vi "Main1.vi"() -> ()   [LabVIEW 2014]
uses:
  Control/Control_process.ctl
  Program Files (x86)/National Instruments/LabVIEW 2018/instr.lib/OSICS 1.1.0/OSICS_LIB.lvlib
  <vilib>/Utility/file.llb/Write Delimited Spreadsheet (string).vi
panel:
  in  "Ref_spec Button":bool
  in  "WL_delay(ms)":u32=800
  in  "Read Button":bool
  in  "VISA_PWM":refnum<visa-resource-name> caption="Power Meter"
  in  "VISA_TLS":refnum<visa-resource-name> caption="Light Source"
  in  "WL_Set":dbl=1310.0 caption="Wavelength"
  in  "PM_delay(ms)":i32=200
  in  "Link Button":bool
  in  "WL_step":dbl=1.0 caption="Step(nm)"
  out "pow_read":dbl caption="Pow"
  in  "Unit(dB:T)":bool
  out "REF?":bool caption="Single Ref."
  out "testing?":bool caption="Bussy"
  out "link?":bool caption="Eq. Online"
  out "Msg":string
  in  "Stop Button":bool
  in  "Sweep Button":bool
  in  "Ref Button":bool
  out "pow_chart":dbl(graph)
  out "WL_Peak":dbl caption="Peak"
  in  "WL_End":dbl=1350.0 caption="End(nm)"
  in  "WL_Start":dbl=1260.0 caption="Start(nm)"
  # "ADDR."
  # "READ"
  # "SWEEP"
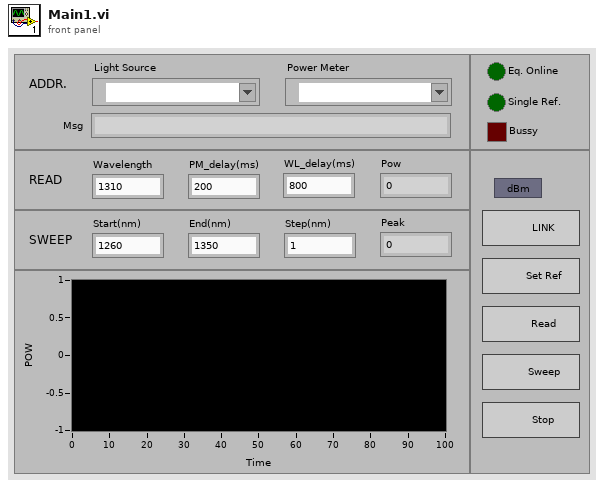
[diagram p1: front panel]
types:
  T1 = typedef "Control_process.ctl" = enum16{"init", "link", "reference", "reference2", "wave_chng", "lockpanel", "single", "sweep", "log_res", "quit"}
  T2 = cluster{"Laser State":bool, "WL/F Value":dbl, "Power (dBm/mW)":dbl, "Power Limit":bool}
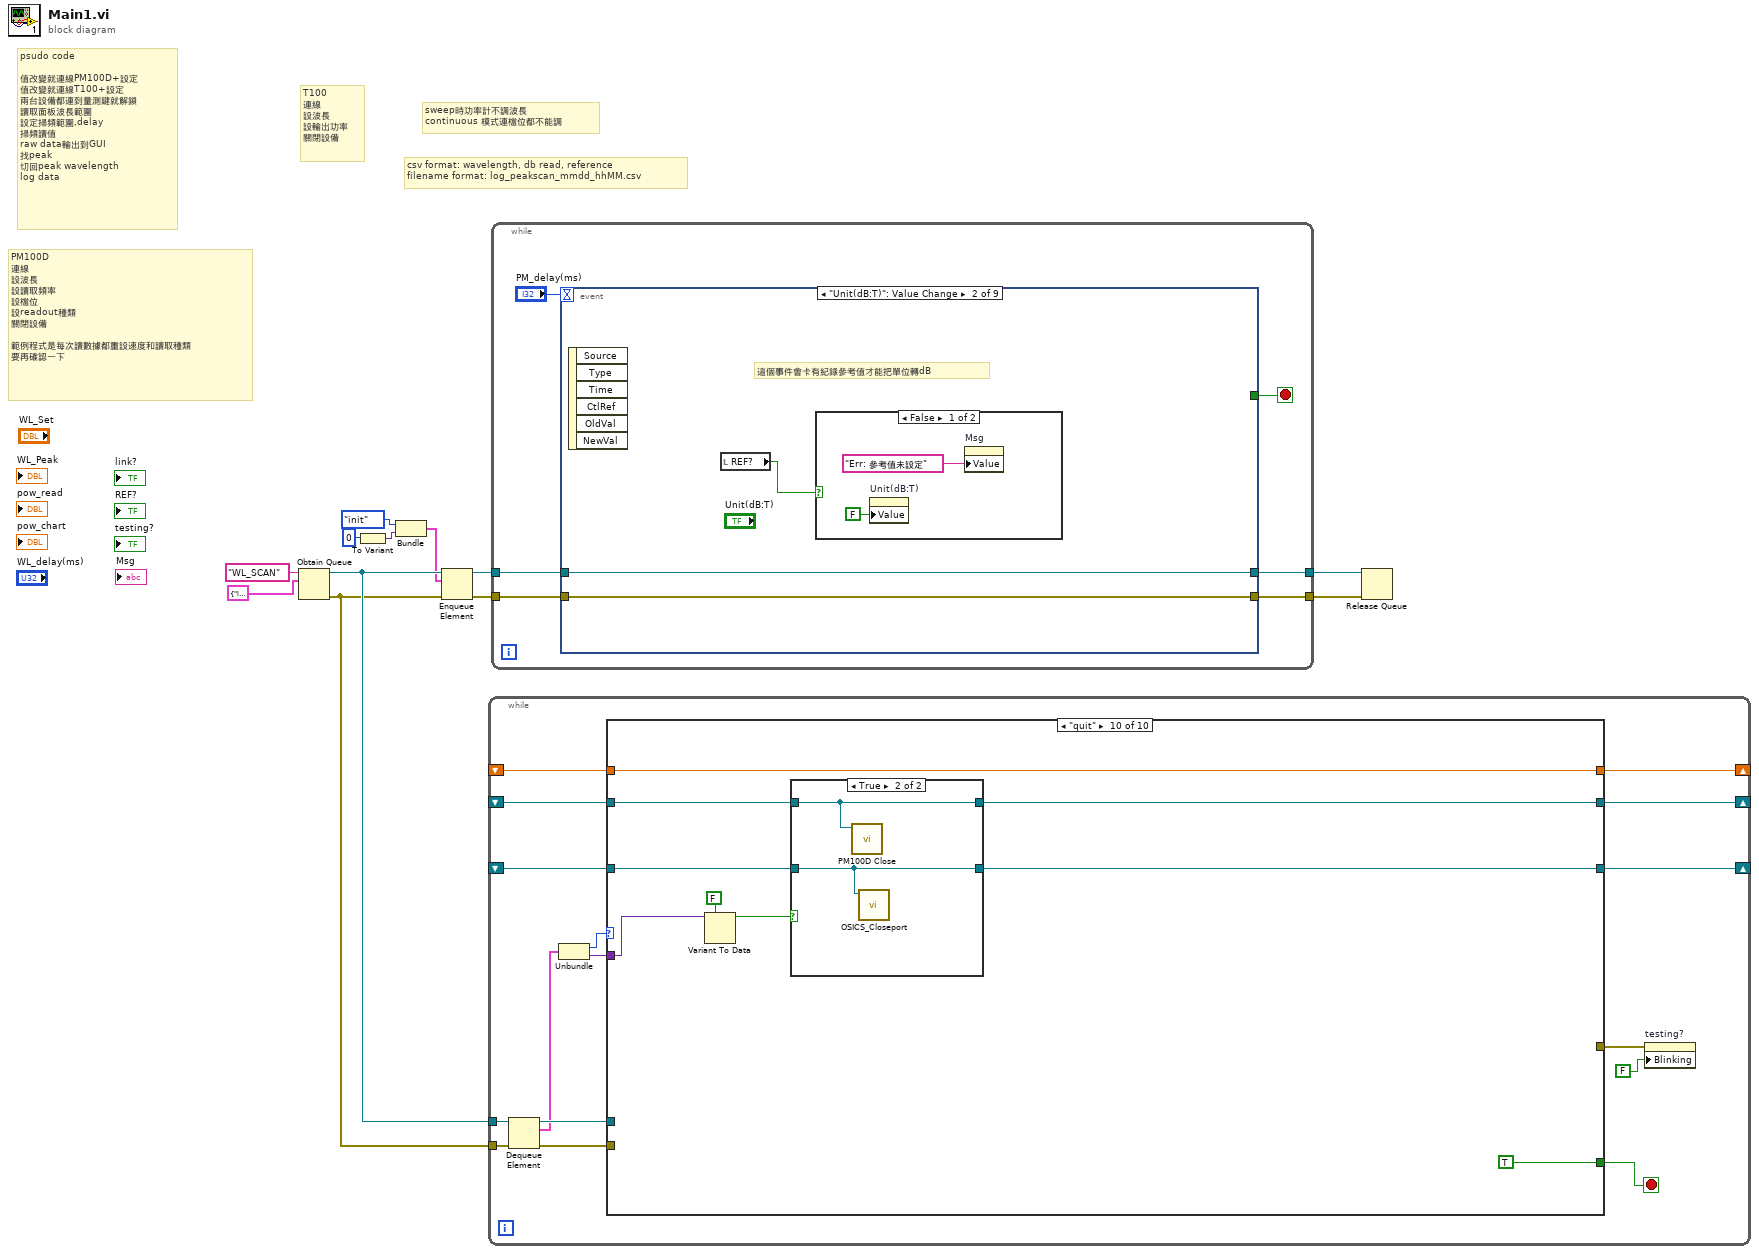
[diagram p0: block diagram]
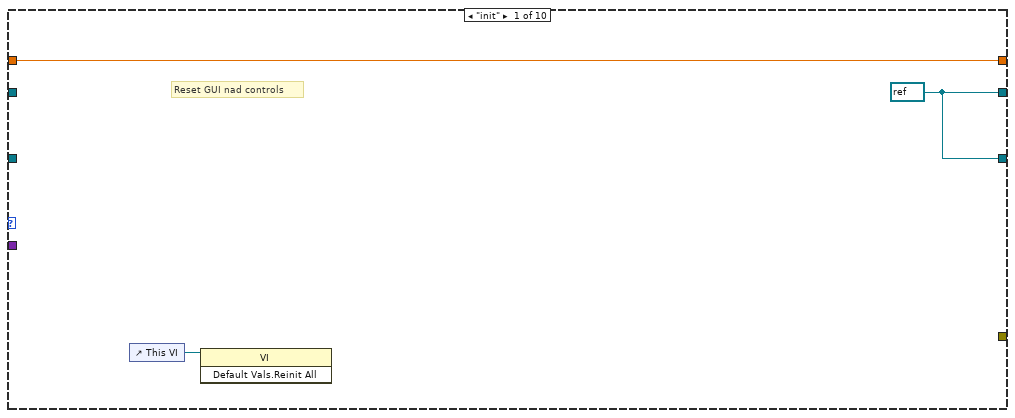
[diagram p2: hidden frame]
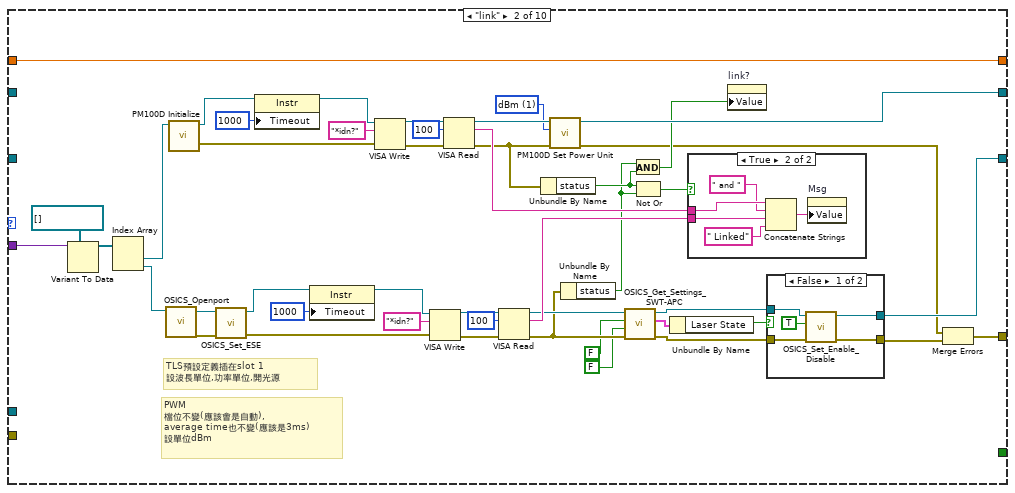
[diagram p3: hidden frame]
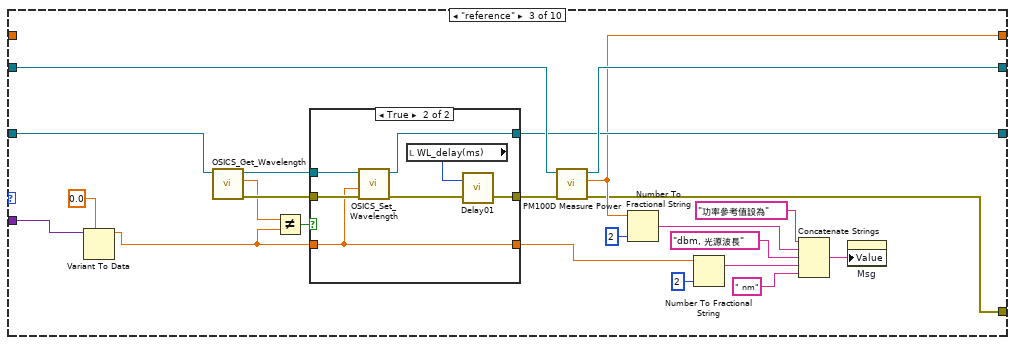
[diagram p6: hidden frame]
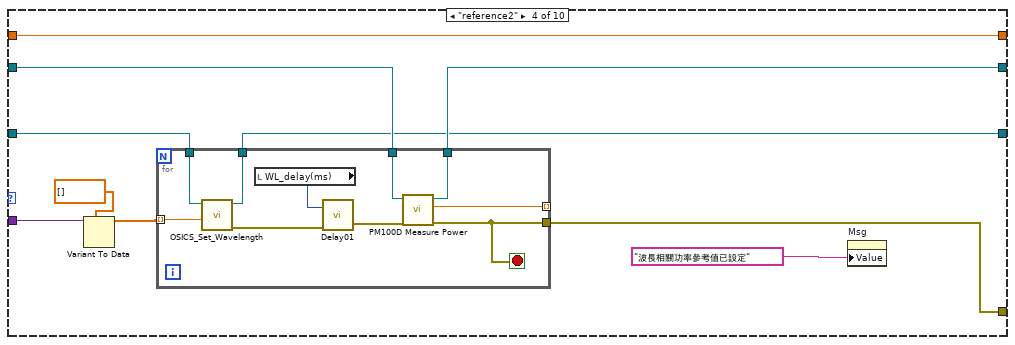
[diagram p8: hidden frame]
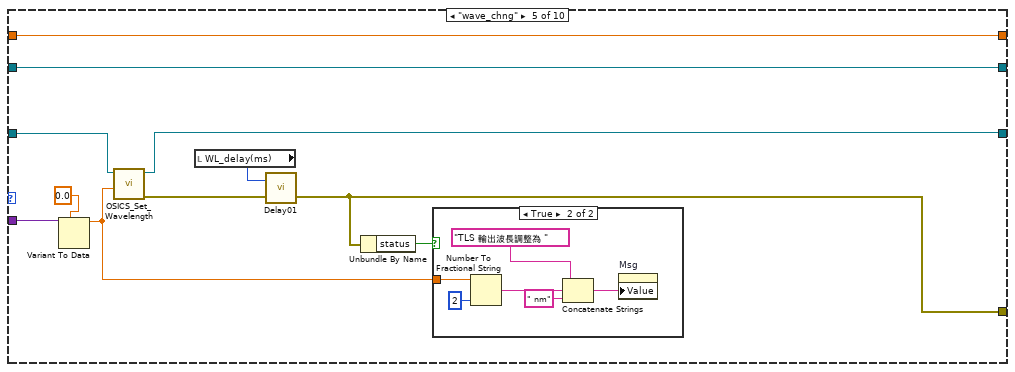
[diagram p9: hidden frame]
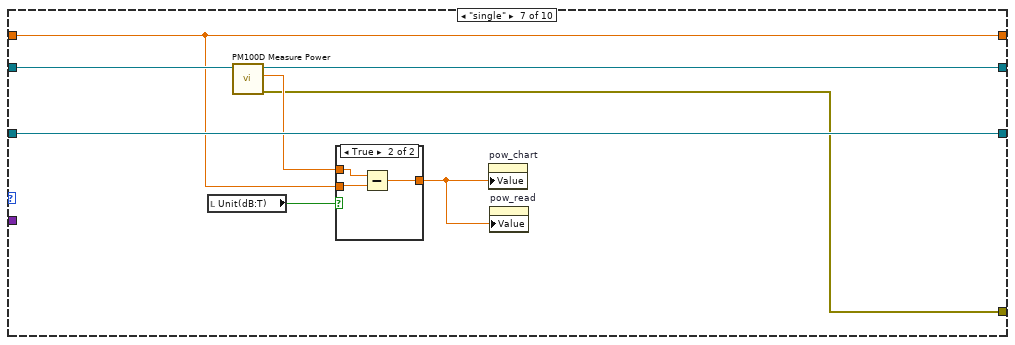
[diagram p12: hidden frame]
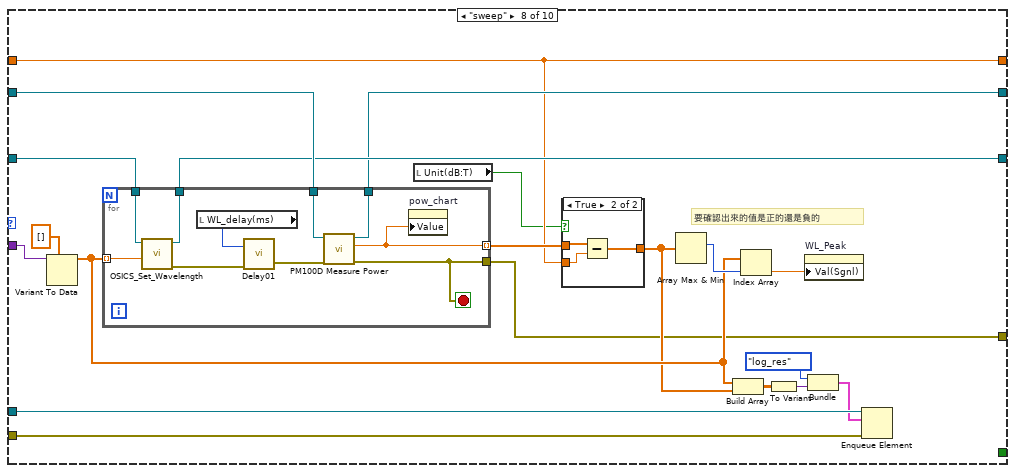
[diagram p14: hidden frame]
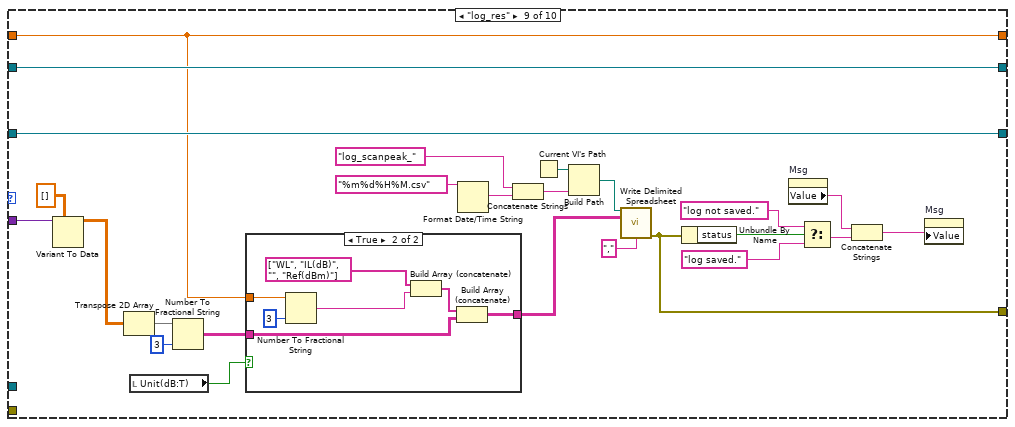
[diagram p16: hidden frame]
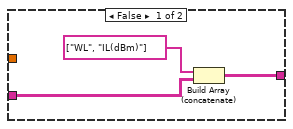
[diagram p17: hidden frame]
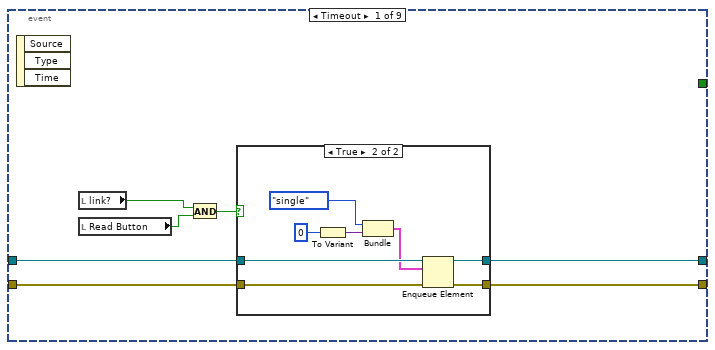
[diagram p19: hidden frame]
diagram:
  # "csv format: wavelength, db read, reference\nfilename format: log_peakscan_mmdd_hhMM.csv"
  # "sweep時功率計不調波長\ncontinuous 模式連檔位都不能調"
  # "T100\n連線\n設波長\n設輸出功率\n關閉設備"
  # "PM100D\n連線\n設波長\n設讀取頻率\n設檔位\n設readout種類\n關閉設備\n\n範例程式是每次讀數據都重設速度和讀取種類\n要再確認一下"
  # "psudo code\n\n值改變就連線PM100D+設定\n值改變就連線T100+設定\n兩台設備都連到量測鍵就解鎖\n讀取面板波長範圍\n設定掃頻範圍,delay\n掃頻讀值\nraw data輸出到GUI\n找peak\n切回peak wavelength\nlog data"
  n1 = Obtain Queue(name (unnamed)="WL_SCAN", element data type=cluster{"Proc":T1, variant} {"Proc"=enum."init", variant}) -> (queue out=w11:refnum<queue>, error out=w6:errorcluster)  [unwired: 3 in, 1 out]
  n2 = To Variant(anything=0) -> (Variant=w3:variant)
  n3 = Bundle("Proc"=Control_process."init", "Variant"=w3) -> (w1:cluster{"Proc":T1, "Variant":variant})  [unwired: 1 in]
  n4 = Enqueue Element(queue=w11, element=w1, error in (no error)=w6) -> (queue out=w7:refnum<queue>, error out=w5:errorcluster)  [unwired: 1 in, 1 out]
  n5 = while {
    tunnel: w6 -> [w26]
    tunnel: w11 -> [w28]
    shift-right: [w17] -> _
    shift-left: _ -> [w21]
    shift-right: [w20] -> _
    shift-left: _ -> [w19]
    shift-right: [w14] -> _
    shift-left: _ -> [w13]
    stop <- w18 stop-if-true
    n6 = Dequeue Element(queue=w28, error in (no error)=w26) -> (queue out=w27:refnum<queue>, element=w24:cluster{"Proc":T1, variant}, error out=w25:errorcluster)  [unwired: 1 in, 1 out]
    n7 = Unbundle(w24) -> ("Proc"=w23:T1, w22:variant)
    n8 = case shown="\"quit\"" w23 {
      tunnel: w27 -> [_ _ _ _ _ _ _ w186 _ _]
      tunnel: w25 -> [_ _ _ _ _ _ _ w185 _ _]
      tunnel: w22 -> [_ w77 w110 w132 w151 _ _ w193 w232 w247]
      tunnel: w21 -> [_ _ w112 w127 w146 w161 w170 w194 w217 w250]
      tunnel: [w31 w43 w108 w125 w152 w160 w169 w192 w228 w248] -> w20
      tunnel: w19 -> [_ _ w106 w128 w153 w160 w169 w191 w228 w252]
      tunnel: [_ _ _ _ _ _ _ _ _ TRUE] -> w18
      tunnel: [w31 w39 w111 w126 w146 w161 w168 w180 w217 w249] -> w17
      tunnel: [_ w33 w92 w124 w143 _ w163 w175 w211 _] -> w15
      tunnel: [w29 w35 w96 w129 w144 w162 w166 w178 w210 w244] -> w14
      tunnel: w13 -> [w29 w35 _ w129 w144 w162 w166 w178 w210 w244]
      frame "init" {
        w31 = refnum<visa-resource-name> refnum ("instrument handle out")
        # "Reset GUI nad controls"
        n9 = control-ref of="This VI"() -> (w30:refnum<vi>)
        n10 = invoke class="VI" method="Default Vals.Reinit All"(reference=w30) -> ()  [unwired: 2 in, 3 out]
      }
      frame "link" {
        w41 = i16 1 items=["Watt", "dBm"] ("Power Unit (Watt)")
        # "TLS預設定義插在slot 1\n設波長單位,功率單位,開光源"
        # "PWM\n檔位不變(應該會是自動), \naverage time也不變(應該是3ms)\n設單位dBm"
        n11 = Variant To Data(type=refnum<visa-resource-name>[] [] ("appended array"), Variant=w77) -> (data=w75:refnum<visa-resource-name>[])  [unwired: 1 in, 1 out]
        n12 = Index Array(array=w75) -> (element #1=w74:refnum<visa-resource-name>, element #2=w64:refnum<visa-resource-name>)  [unwired: 2 in]
        n13 = call "OSICS_Openport.vi"("VISA IN"=w64) -> ("error out"=w65:errorcluster, "VISA OUT"=w63:refnum<visa-resource-name>)  [unwired: 9 in]
        n14 = call "PM100D Initialize.vi"("resource name"=w74) -> ("error out"=w69:errorcluster, "instrument handle out"=w68:refnum<visa-resource-name>)  [unwired: 9 in]
        n15 = call "OSICS_Set_ESE.vi"("error in (no error)"=w65, "VISA resource name"=w63) -> ("error out"=w56:errorcluster, "VISA resource name out"=w55:refnum<visa-resource-name>)  [unwired: 8 in]
        n16 = property class="Instr"(reference=w68, "Timeout"=u32 1000 ("General Settings:Timeout Value")) -> (reference out=w67:refnum<visa-resource-name>)  [unwired: 1 in, 1 out]
        n17 = property class="Instr"(reference=w55, "Timeout"=u32 1000 ("General Settings:Timeout Value")) -> (reference out=w61:refnum<visa-resource-name>)  [unwired: 1 in, 1 out]
        n18 = VISA Write(VISA resource name=w67, write buffer="*idn?", error in (no error)=w69) -> (VISA resource name out=w71:refnum<visa-resource-name>, error out=w73:errorcluster)  [unwired: 1 out]
        n19 = VISA Write(VISA resource name=w61, write buffer="*idn?", error in (no error)=w56) -> (VISA resource name out=w59:refnum<visa-resource-name>, error out=w57:errorcluster)  [unwired: 1 out]
        n20 = VISA Read(VISA resource name=w71, byte count=u32 100, error in (no error)=w73) -> (VISA resource name out=w42:refnum<visa-resource-name>, read buffer=w53:string, error out=w40:errorcluster)  [unwired: 1 out]
        n21 = VISA Read(VISA resource name=w59, byte count=u32 100, error in (no error)=w57) -> (VISA resource name out=w51:refnum<visa-resource-name>, read buffer=w54:string, error out=w48:errorcluster)  [unwired: 1 out]
        n22 = Unbundle By Name(w40) -> ("status"=w37:bool)
        n23 = call "PM100D Set Power Unit.vi"("error in (no error)"=w40, "Power Unit (Watt)"=w41, "instrument handle"=w42) -> ("error out"=w32:errorcluster, "instrument handle out"=w39:refnum<visa-resource-name>)  [unwired: 7 in]
        n24 = Unbundle By Name(w48) -> ("status"=w36:bool)
        n25 = call "OSICS_Get_Settings_SWT-APC.vi"("error in"=w48, "Power Unit(dBm/mW)"=FALSE, "WL/F unit (nm/GHz)"=FALSE, "VISA IN"=w51) -> ("error out"=w44:errorcluster, "Laser Settings (Cluster)"=w50:T2, "VISA OUT"=w45:refnum<visa-resource-name>)  [unwired: 5 in]
        n26 = And(x=w36, y=w37) -> (x .and. y?=w38:bool)
        n27 = Not Or(1:w36, 2:w37) -> (0:w52:bool)
        n28 = Unbundle By Name(w50) -> ("Laser State"=w49:bool)
        n29 = case shown="True" w52 {
          tunnel: w54 -> [_ w89]
          tunnel: w53 -> [_ w88]
          frame False {
          }
          frame True {
            n30 = Concatenate Strings(w88, " and " ("string"), w89, " Linked" ("string")) -> (w86:string)
            n31 = property on="Msg" class="Str"("Value"=w86) -> ()  [unwired: 2 in, 2 out]
          }
        }
        n32 = property on="link?" class="Bool (strict)"("Value"=w38) -> ()  [unwired: 2 in, 2 out]
        n33 = case shown="False" w49 {
          tunnel: w45 -> [w81 w84]
          tunnel: w44 -> [w80 w83]
          tunnel: [w79 w84] -> w43
          tunnel: [w78 w83] -> w34
          frame False {
            n34 = call "OSICS_Set_Enable_Disable.vi"("error in"=w80, "Laser State (False:DISABLED)"=TRUE, "VISA IN"=w81) -> ("error out"=w78:errorcluster, "VISA OUT"=w79:refnum<visa-resource-name>)  [unwired: 6 in, 1 out]
          }
          frame True {
          }
        }
        n35 = Merge Errors(w32, w34) -> (w33:errorcluster)
      }
      frame "reference" {
        n36 = Variant To Data(type=0.0, Variant=w110) -> (data=w90:dbl)  [unwired: 1 in, 1 out]
        n37 = call "OSICS_Get_Wavelength.vi"("VISA IN"=w106) -> ("error out"=w105:errorcluster, "WL/Frequency Value"=w103:dbl, "VISA OUT"=w107:refnum<visa-resource-name>)  [unwired: 7 in, 1 out]
        n38 = Not Equal?(x=w103, y=w90) -> (x != y?=w104:bool)
        n39 = case shown="True" w104 {
          tunnel: [w114 w120] -> w109
          tunnel: [w115 w119] -> w108
          tunnel: w107 -> [w115 w118]
          tunnel: w105 -> [w114 w117]
          tunnel: w90 -> [w113 w116]
          tunnel: [w113 w116] -> w93
          frame False {
          }
          frame True {
            n40 = call "OSICS_Set_Wavelength.vi"("error in"=w117, "WL/Frequency Value"=w116, "VISA IN"=w118) -> ("error out"=w122:errorcluster, "VISA OUT"=w119:refnum<visa-resource-name>)  [unwired: 6 in, 1 out]
            n41 = local read "WL_delay(ms)"() -> (w121:u32)
            n42 = call "Delay01.vi"("error in"=w122, "ms delay"=w121) -> ("error out"=w120:errorcluster)  [unwired: 1 in]
          }
        }
        n43 = call "PM100D Measure Power.vi"("error in (no error)"=w109, "instrument handle"=w112) -> ("error out"=w92:errorcluster, "Power"=w96:dbl, "instrument handle out"=w111:refnum<visa-resource-name>)  [unwired: 7 in]
        n44 = Number To Fractional String(number=w96, precision (6)=i16 2) -> (F-format string=w95:string)  [unwired: 2 in]
        n45 = Number To Fractional String(number=w93, precision (6)=i16 2) -> (F-format string=w100:string)  [unwired: 2 in]
        n46 = Concatenate Strings("功率參考值設為" ("string"), w95, "dbm, 光源波長" ("string"), w100, " nm" ("string")) -> (w99:string)
        n47 = property on="Msg" class="Str"("Value"=w99) -> ()  [unwired: 2 in, 2 out]
      }
      frame "reference2" {
        n48 = Variant To Data(type=dbl[] [], Variant=w132) -> (data=w130:dbl[])  [unwired: 1 in, 1 out]
        n49 = for {
          tunnel: w127 -> [w142]
          tunnel: [w141] -> w126
          tunnel: [w138] -> w125
          tunnel: w128 -> [w137]
          tunnel: [w134] -> w124
          tunnel: [w136] -> _ mode=indexing
          tunnel: w130 -> [w135] mode=indexing
          stop <- w134 stop-if-true
          n50 = call "OSICS_Set_Wavelength.vi"("WL/Frequency Value"=w135, "VISA IN"=w137) -> ("error out"=w140:errorcluster, "VISA OUT"=w138:refnum<visa-resource-name>)  [unwired: 7 in, 1 out]
          n51 = local read "WL_delay(ms)"() -> (w133:u32)
          n52 = call "Delay01.vi"("error in"=w140, "ms delay"=w133) -> ("error out"=w139:errorcluster)  [unwired: 1 in]
          n53 = call "PM100D Measure Power.vi"("error in (no error)"=w139, "instrument handle"=w142) -> ("error out"=w134:errorcluster, "Power"=w136:dbl, "instrument handle out"=w141:refnum<visa-resource-name>)  [unwired: 7 in]
        }
        n54 = property on="Msg" class="Str"("Value"="波長相關功率參考值已設定" ("string")) -> ()  [unwired: 2 in, 2 out]
      }
      frame "wave_chng" {
        n55 = Variant To Data(type=0.0, Variant=w151) -> (data=w145:dbl)  [unwired: 1 in, 1 out]
        n56 = call "OSICS_Set_Wavelength.vi"("WL/Frequency Value"=w145, "VISA IN"=w153) -> ("error out"=w149:errorcluster, "VISA OUT"=w152:refnum<visa-resource-name>)  [unwired: 7 in, 1 out]
        n57 = local read "WL_delay(ms)"() -> (w147:u32)
        n58 = call "Delay01.vi"("error in"=w149, "ms delay"=w147) -> ("error out"=w143:errorcluster)  [unwired: 1 in]
        n59 = Unbundle By Name(w143) -> ("status"=w148:bool)
        n60 = case shown="True" w148 {
          tunnel: w145 -> [_ w156]
          frame False {
          }
          frame True {
            n61 = Number To Fractional String(number=w156, precision (6)=i16 2) -> (F-format string=w155:string)  [unwired: 2 in]
            n62 = Concatenate Strings("TLS 輸出波長調整為 " ("Msg"), w155, " nm" ("string")) -> (w159:string)
            n63 = property on="Msg" class="Str"("Value"=w159) -> ()  [unwired: 2 in, 2 out]
          }
        }
      }
      frame "lockpanel" {
      }
      frame "single" {
        n64 = local read "Unit(dB:T)"() -> (w164:bool)
        n65 = call "PM100D Measure Power.vi"("instrument handle"=w170) -> ("error out"=w163:errorcluster, "Power"=w167:dbl, "instrument handle out"=w168:refnum<visa-resource-name>)  [unwired: 8 in]
        n66 = case shown="True" w164 {
          tunnel: w167 -> [w171 w174]
          tunnel: w166 -> [_ w173]
          tunnel: [w171 w172] -> w165
          frame False {
          }
          frame True {
            n67 = Subtract(x=w174, y=w173) -> (x-y=w172:dbl)
          }
        }
        n68 = property on="pow_chart" class="WFChart (strict)"("Value"=w165) -> ()  [unwired: 2 in, 2 out]
        n69 = property on="pow_read" class="DigNum (strict)"("Value"=w165) -> ()  [unwired: 2 in, 2 out]
      }
      frame "sweep" {
        # "要確認出來的值是正的還是負的"
        n70 = Variant To Data(type=dbl[] [], Variant=w193) -> (data=w187:dbl[])  [unwired: 1 in, 1 out]
        n71 = for {
          tunnel: w194 -> [w208]
          tunnel: [w207] -> w180
          tunnel: [w203] -> w192
          tunnel: w191 -> [w202]
          tunnel: [w199] -> w175
          tunnel: [w201] -> w179 mode=indexing
          tunnel: w187 -> [w200] mode=indexing
          stop <- w199 stop-if-true
          n72 = call "OSICS_Set_Wavelength.vi"("WL/Frequency Value"=w200, "VISA IN"=w202) -> ("error out"=w206:errorcluster, "VISA OUT"=w203:refnum<visa-resource-name>)  [unwired: 7 in, 1 out]
          n73 = local read "WL_delay(ms)"() -> (w205:u32)
          n74 = call "Delay01.vi"("error in"=w206, "ms delay"=w205) -> ("error out"=w204:errorcluster)  [unwired: 1 in]
          n75 = call "PM100D Measure Power.vi"("error in (no error)"=w204, "instrument handle"=w208) -> ("error out"=w199:errorcluster, "Power"=w201:dbl, "instrument handle out"=w207:refnum<visa-resource-name>)  [unwired: 7 in]
          n76 = property on="pow_chart" class="WFChart (strict)"("Value"=w201) -> ()  [unwired: 2 in, 2 out]
        }
        n77 = local read "Unit(dB:T)"() -> (w176:bool)
        n78 = case shown="True" w176 {
          tunnel: w179 -> [w195 w198]
          tunnel: w178 -> [_ w197]
          tunnel: [w195 w196] -> w177
          frame False {
          }
          frame True {
            n79 = Subtract(x=w198, y=w197) -> (x-y=w196:dbl[])
          }
        }
        n80 = Array Max & Min(array=w177) -> (max index (indices)=w189:i32)  [unwired: 3 out]
        n81 = Build Array(w187, w177) -> (w182:dbl[][])
        n82 = Index Array(array=w187, index=w189) -> (element=w188:dbl)
        n83 = To Variant(anything=w182) -> (Variant=w183:variant)
        n84 = property on="WL_Peak" class="DigNum (strict)"("Val(Sgnl)"=w188) -> ()  [unwired: 2 in, 2 out]
        n85 = Bundle("Proc"=Control_process."log_res", "Variant"=w183) -> (w181:cluster{"Proc":T1, "Variant":variant})  [unwired: 1 in]
        n86 = Enqueue Element(queue=w186, element=w181, error in (no error)=w185) -> ()  [unwired: 1 in, 3 out]
      }
      frame "log_res" {
        n87 = Variant To Data(type=dbl[][] [] ("appended array"), Variant=w232) -> (data=w214:dbl[][])  [unwired: 1 in, 1 out]
        n88 = Transpose 2D Array(2D array=w214) -> (transposed array=w215:dbl[][])
        n89 = local read "Unit(dB:T)"() -> (w209:bool)
        n90 = Number To Fractional String(number=w215, precision (6)=i16 3) -> (F-format string=w213:string[][])  [unwired: 2 in]
        n91 = case shown="True" w209 {
          tunnel: w213 -> [w236 w243]
          tunnel: [w234 w242] -> w212
          tunnel: w210 -> [_ w239]
          frame False {
            n92 = Build Array (concatenate)(string[] ["WL", "IL(dBm)"], w236) -> (w234:string[][])
          }
          frame True {
            n93 = Number To Fractional String(number=w239, precision (6)=i16 3) -> (F-format string=w238:string)  [unwired: 2 in]
            n94 = Build Array (concatenate)(string[] ["WL", "IL(dB)", "", "Ref(dBm)"], w238) -> (w241:string[])
            n95 = Build Array (concatenate)(w241, w243) -> (w242:string[][])
          }
        }
        n96 = Format Date/Time String(time format string (%c)="%m%d%H%M.csv") -> (date/time string=w225:string)  [unwired: 2 in]
        n97 = Concatenate Strings("log_scanpeak_" ("string"), w225) -> (w224:string)
        n98 = Current VI's Path() -> (path=w230:path)
        n99 = Build Path(base path=w230, name or relative path=w224) -> (appended path=w229:path)
        n100 = call-poly <vilib>:"Write Delimited Spreadsheet.vi"("file path (dialog if empty)"=w229, "2D data"=w212, "delimiter (\\t)"="," ("delimiter (\\t)")) -> ("error out"=w211:errorcluster)  [unwired: 11 in, 1 out]
        n101 = Unbundle By Name(w211) -> ("status"=w223:bool)
        n102 = property on="Msg" class="Str"() -> ("Value"=w220:string)  [unwired: 2 in, 2 out]
        n103 = Select(t="log not saved.", s=w223, f="log saved.") -> (s? t:f=w221:string)
        n104 = Concatenate Strings(w220, w221) -> (w222:string)
        n105 = property on="Msg" class="Str"("Value"=w222) -> ()  [unwired: 2 in, 2 out]
      }
      frame "quit" {
        n106 = Variant To Data(type=FALSE, Variant=w247) -> (data=w245:bool)  [unwired: 1 in, 1 out]
        n107 = case shown="True" w245 {
          tunnel: w252 -> [w253 w255]
          tunnel: w250 -> [w254 w256]
          tunnel: [w254 w256] -> w249
          tunnel: [w253 w255] -> w248
          frame False {
          }
          frame True {
            n108 = call "PM100D Close.vi"("instrument handle"=w256) -> ()  [unwired: 10 in, 1 out]
            n109 = call "OSICS_Closeport.vi"("VISA IN"=w255) -> ()  [unwired: 10 in, 1 out]
          }
        }
      }
    }
    n110 = property on="testing?" class="Bool (strict)"(error in=w15, "Blinking"=FALSE) -> ()  [unwired: 1 in, 2 out]
  }
  n111 = while {
    tunnel: w7 -> [w260]
    tunnel: w5 -> [w261]
    tunnel: [w259] -> w10
    tunnel: [w258] -> w9
    stop <- w262 stop-if-true
    n112 = event shown="[1] \"Unit(dB:T)\": Value Change" {
      selector: _ -> [_ _ _ _ _ _ _ _ _]
      dyn-events: _ -> [_ _ _ _ _ _ _ _ _]
      timeout: "PM_delay(ms)" -> [_ _ _ _ _ _ _ _ _]
      tunnel: [_ _ _ _ _ _ _ _ TRUE] -> w262
      tunnel: w261 -> [w268 w281 w289 w310 w326 w342 w349 w378 w400]
      tunnel: w260 -> [w269 w282 w290 w311 w327 w343 w351 w381 w398]
      tunnel: [w267 w282 w288 w309 w325 w343 w350 w380 w397] -> w259
      tunnel: [w266 w281 w287 w308 w324 w342 w348 w379 w399] -> w258
      event Timeout {
        n113 = event-data() -> ()  [unwired: 1 in, 3 out]
        n114 = local read "link?"() -> (w263:bool)
        n115 = local read "Read Button"() -> (w264:bool)
        n116 = And(x=w263, y=w264) -> (x .and. y?=w265:bool)
        n117 = case shown="True" w265 {
          tunnel: w269 -> [w271 w279]
          tunnel: w268 -> [w270 w278]
          tunnel: [w271 w277] -> w267
          tunnel: [w270 w276] -> w266
          frame False {
          }
          frame True {
            n118 = To Variant(anything=0) -> (Variant=w275:variant)
            n119 = Bundle("Proc"=Control_process."single", "Variant"=w275) -> (w273:cluster{"Proc":T1, "Variant":variant})  [unwired: 1 in]
            n120 = Enqueue Element(queue=w279, element=w273, error in (no error)=w278) -> (queue out=w277:refnum<queue>, error out=w276:errorcluster)  [unwired: 1 in, 1 out]
          }
        }
      }
      event "Unit(dB:T)": Value Change {
        # "這個事件會卡有紀錄參考值才能把單位轉dB"
        n121 = event-data() -> ()  [unwired: 1 in, 6 out]
        n122 = local read "REF?"() -> (w280:bool)
        n123 = case shown="False" w280 {
          frame False {
            n124 = property on="Unit(dB:T)" class="Bool (strict)"("Value"=FALSE ("Unit")) -> ()  [unwired: 2 in, 2 out]
            n125 = property on="Msg" class="Str"("Value"="Err: 參考值未設定" ("Msg")) -> ()  [unwired: 2 in, 2 out]
          }
          frame True {
          }
        }
      }
      event "Link Button": Value Change {
        n126 = event-data() -> ()  [unwired: 1 in, 1 out]
        n127 = Empty String/Path?(string/path="VISA_PWM") -> (empty?=w292:bool)
        n128 = Empty String/Path?(string/path="VISA_TLS") -> (empty?=w293:bool)
        n129 = Not Or(1:w292, 2:w293) -> (0:w291:bool)
        n130 = case shown="False" w291 {
          tunnel: w290 -> [w296 w306]
          tunnel: w289 -> [w295 w305]
          tunnel: [w296 w304] -> w288
          tunnel: [w295 w303] -> w287
          tunnel: "VISA_TLS" -> [_ w300]
          tunnel: "VISA_PWM" -> [_ w299]
          frame False {
            n131 = property on="Msg" class="Str"("Value"="Err: 未選擇儀器位址" ("Msg")) -> ()  [unwired: 2 in, 2 out]
          }
          frame True {
            n132 = Build Array(w300, w299) -> (w298:refnum<visa-resource-name>[])
            n133 = To Variant(anything=w298) -> (Variant=w297:variant)
            n134 = Bundle("Proc"=Control_process."link", "Variant"=w297) -> (w301:cluster{"Proc":T1, "Variant":variant})  [unwired: 1 in]
            n135 = Enqueue Element(queue=w306, element=w301, error in (no error)=w305) -> (queue out=w304:refnum<queue>, error out=w303:errorcluster)  [unwired: 1 in, 1 out]
          }
        }
      }
      event "Ref Button": Value Change {
        n136 = event-data() -> ()  [unwired: 1 in, 6 out]
        n137 = local read "link?"() -> (w307:bool)
        n138 = case shown="True" w307 {
          tunnel: w311 -> [w314 w322]
          tunnel: w310 -> [w313 w321]
          tunnel: [w314 w320] -> w309
          tunnel: [w313 w319] -> w308
          frame False {
            n139 = property on="Msg" class="Str"("Value"="Err: 設備未連結" ("Msg")) -> ()  [unwired: 2 in, 2 out]
          }
          frame True {
            n140 = local read "WL_Set"() -> (w315:dbl)
            n141 = To Variant(anything=w315) -> (Variant=w318:variant)
            n142 = Bundle("Proc"=Control_process."reference", "Variant"=w318) -> (w316:cluster{"Proc":T1, "Variant":variant})  [unwired: 1 in]
            n143 = Enqueue Element(queue=w322, element=w316, error in (no error)=w321) -> (queue out=w320:refnum<queue>, error out=w319:errorcluster)  [unwired: 1 in, 1 out]
          }
        }
      }
      event "Ref_spec Button": Value Change {
        n144 = event-data() -> ()  [unwired: 1 in, 6 out]
        n145 = local read "link?"() -> (w323:bool)
        n146 = case shown="True" w323 {
          tunnel: w327 -> [w330 w338]
          tunnel: w326 -> [w329 w337]
          tunnel: [w330 w336] -> w325
          tunnel: [w329 w335] -> w324
          frame False {
            n147 = property on="Msg" class="Str"("Value"="Err: 設備未連結" ("Msg")) -> ()  [unwired: 2 in, 2 out]
          }
          frame True {
            n148 = local read "WL_Set"() -> (w331:dbl)
            n149 = To Variant(anything=w331) -> (Variant=w334:variant)
            n150 = Bundle("Proc"=Control_process."reference", "Variant"=w334) -> (w332:cluster{"Proc":T1, "Variant":variant})  [unwired: 1 in]
            n151 = Enqueue Element(queue=w338, element=w332, error in (no error)=w337) -> (queue out=w336:refnum<queue>, error out=w335:errorcluster)  [unwired: 1 in, 1 out]
          }
        }
      }
      event "Read Button": Value Change {
        n152 = event-data() -> ()  [unwired: 1 in, 6 out]
        n153 = local read "link?"() -> (w340:bool)
        n154 = And(x=w340, y="Read Button") -> (x .and. y?=w339:bool)
        n155 = case shown="True" w339 {
          selector: w339 -> [w345 w346]
          frame False {
            n156 = property on="Read Button" class="Bool (strict)"("Value"=w345) -> ()  [unwired: 2 in, 2 out]
            n157 = property on="Msg" class="Str"("Value"="Err: 設備未連結" ("Msg")) -> ()  [unwired: 2 in, 2 out]
          }
          frame True {
            n158 = property on="testing?" class="Bool (strict)"("Blinking"=w346) -> ()  [unwired: 2 in, 2 out]
          }
        }
      }
      event "Sweep Button": Value Change {
        n159 = event-data() -> ()  [unwired: 1 in, 1 out]
        n160 = local read "link?"() -> (w347:bool)
        n161 = case shown="True" w347 {
          tunnel: w351 -> [w354 w366]
          tunnel: [w354 w365] -> w350
          tunnel: w349 -> [w353 w362]
          tunnel: [w353 w361] -> w348
          frame False {
            n162 = property on="Msg" class="Str"("Value"="Err: 設備未連結" ("Msg")) -> ()  [unwired: 2 in, 2 out]
          }
          frame True {
            n163 = while {
              tunnel: "WL_step" -> [w371]
              tunnel: "WL_End" -> [w370]
              shift-right: [w372] -> _
              shift-left: "WL_Start" -> [w373]
              tunnel: [w373] -> w357 mode=indexing
              i -> [w369]
              stop <- w368 stop-if-true
              # "掃描點"
              n164 = Add(x=w373, y=w371) -> (x+y=w372:dbl)
              n165 = Greater?(x=w372, y=w370) -> (0:w375:bool)
              n166 = Equal?(x=9999, y=w369) -> (x = y?=w374:bool)
              n167 = Or(x=w375, y=w374) -> (x .or. y?=w368:bool)
            }
            n168 = To Variant(anything=w357) -> (Variant=w364:variant)
            n169 = Bundle("Proc"=Control_process."sweep", "Variant"=w364) -> (w363:cluster{"Proc":T1, "Variant":variant})  [unwired: 1 in]
            n170 = Enqueue Element(queue=w366, element=w363, error in (no error)=w362) -> (queue out=w365:refnum<queue>, error out=w361:errorcluster)  [unwired: 1 in, 1 out]
            n171 = property on="testing?" class="Bool (strict)"("Blinking"=TRUE) -> ()  [unwired: 2 in, 2 out]
            n172 = property on="Msg" class="Str"("Value"="波長掃描中......" ("Msg")) -> ()  [unwired: 2 in, 2 out]
          }
        }
      }
      event "WL_Set", "WL_Peak": Value Change {
        n173 = event-data() -> ("NewVal"=w382:dbl)  [unwired: 1 in]
        n174 = local read "link?"() -> (w377:bool)
        n175 = case shown="True" w377 {
          tunnel: w382 -> [_ w391]
          tunnel: w381 -> [w384 w389]
          tunnel: [w384 w388] -> w380
          tunnel: [w383 w387] -> w379
          tunnel: w378 -> [w383 w386]
          frame False {
          }
          frame True {
            n176 = To Variant(anything=w391) -> (Variant=w392:variant)
            n177 = Bundle("Proc"=Control_process."wave_chng", "Variant"=w392) -> (w385:cluster{"Proc":T1, "Variant":variant})  [unwired: 1 in]
            n178 = Enqueue Element(queue=w389, element=w385, error in (no error)=w386) -> (queue out=w388:refnum<queue>, error out=w387:errorcluster)  [unwired: 1 in, 1 out]
          }
        }
      }
      event "Stop Button": Value Change; Panel Close {
        n179 = event-data() -> ()  [unwired: 1 in, 3 out]
        n180 = local read "link?"() -> (w393:bool)
        n181 = To Variant(anything=w393) -> (Variant=w395:variant)
        n182 = Bundle("Proc"=Control_process."quit", "Variant"=w395) -> (w394:cluster{"Proc":T1, "Variant":variant})  [unwired: 1 in]
        n183 = Enqueue Element At Opposite End(queue=w398, element=w394, error in (no error)=w400) -> (queue out=w397:refnum<queue>, error out=w399:errorcluster)  [unwired: 1 in, 1 out]
      }
    }
  }
  n184 = Release Queue(queue=w10, error in (no error)=w9) -> ()  [unwired: 1 in, 3 out]
